vi "AccessBuiltInProperties.vi"(11 "Sequence Context In":refnum<k7>) -> (0 "error out":errorcluster, 1 "Execution Time":dbl, 2 "Number of Steps":i32, 3 "Sequence Name":string)   [LabVIEW 2011]
doc: "This VI demonstrates how to access Built-in TestStand properties and methods."
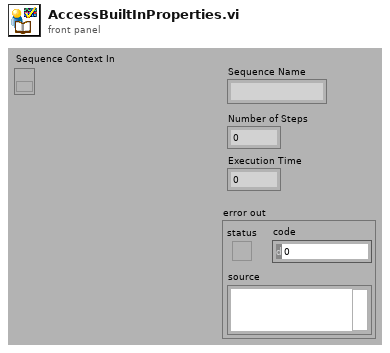
[diagram p1: front panel]
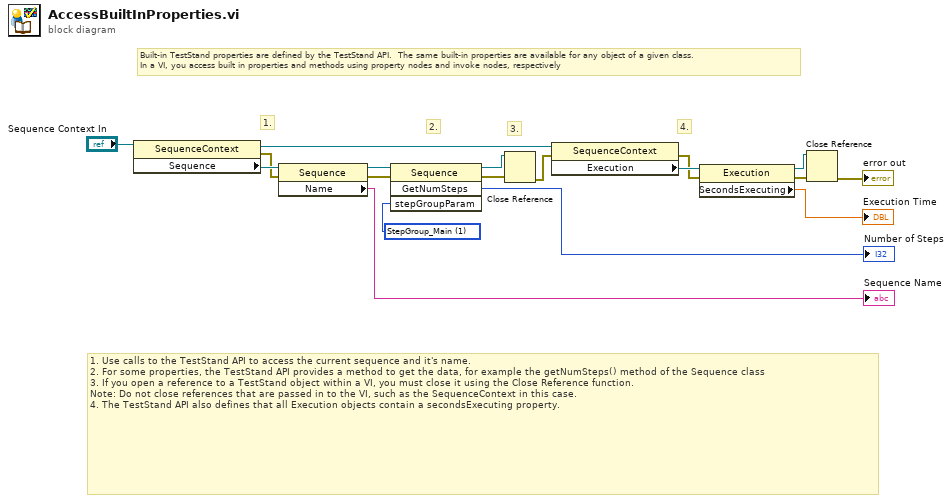
[diagram p0: block diagram]
diagram:
  w10 = 1 items=["StepGroup_Setup", "StepGroup_Main", "StepGroup_Cleanup"] ("stepGroupParam")
  # "Built-in TestStand properties are defined by the TestStand API.  The same built-in properties are available for any object of a given class.\nIn a VI, you access built in properties and methods using property nodes and invoke nodes, respectively"
  # "4."
  # "3."
  # "2."
  # "1."
  # "1. Use calls to the TestStand API to access the current sequence and it's name.\n2. For some properties, the TestStand API provides a method to get the data, for example the getNumSteps() method of the Sequence class\n3. If you open a reference to a TestStand object within a VI, you must close it using the Close Reference function.  \nNote: Do not close references that are passed in to the VI, such as the SequenceContext in this case. \n4. The TestStand API also defines that all Execution objects contain a secondsExecuting property."
  n1 = property class="SequenceContext"(reference="Sequence Context In") -> (reference out=w15:refnum<k7>, error out=w16:errorcluster, "Sequence"=w17:refnum<k7>)  [unwired: 1 in]
  n2 = property class="Sequence"(reference=w17, error in=w16) -> (reference out=w11:refnum<k7>, error out=w12:errorcluster, "Name"=→"Sequence Name":string)
  n3 = invoke class="Sequence" method="GetNumSteps"(reference=w11, error in=w12, "stepGroupParam"=w10) -> (reference out=w8:refnum<k7>, error out=w9:errorcluster, "GetNumSteps"=→"Number of Steps":i32)  [unwired: 1 in, 1 out]
  n4 = Close Reference(reference=w8, error in (no error)=w9) -> (error out=w7:errorcluster)
  n5 = property class="SequenceContext"(reference=w15, error in=w7) -> (error out=w13:errorcluster, "Execution"=w14:refnum<k7>)  [unwired: 1 out]
  n6 = property class="Execution"(reference=w14, error in=w13) -> (reference out=w5:refnum<k7>, error out=w6:errorcluster, "SecondsExecuting"=→"Execution Time":dbl)
  n7 = Close Reference(reference=w5, error in (no error)=w6) -> (error out=→"error out":errorcluster)
